vi "Flatten2DValues.vi"(9 "NumValues":u16[](array[numeric])=[1, 1, 1, 2, 4, 1], 10 "Values 2D":dbl[][](array[numeric])=[[1712710454.0, 9999.0], [0.0, 9999.0], [0.0, 9999.0], [1.0, 2.0], [9999.0, 9999.0], [9999.0, 9999.0]] format="%.2f", 11 "NumFrames":i32=6) -> (2 "Values 1D":dbl[](array[numeric]) format="%.2f")   [LabVIEW 2024]
panel:
  # "Takes a 2D array of values and flattens it to 1D.  Removes or adds extra\nelements based on NumValues.  The result is a 1D Values array of the\nexact size to hold all write and read data."
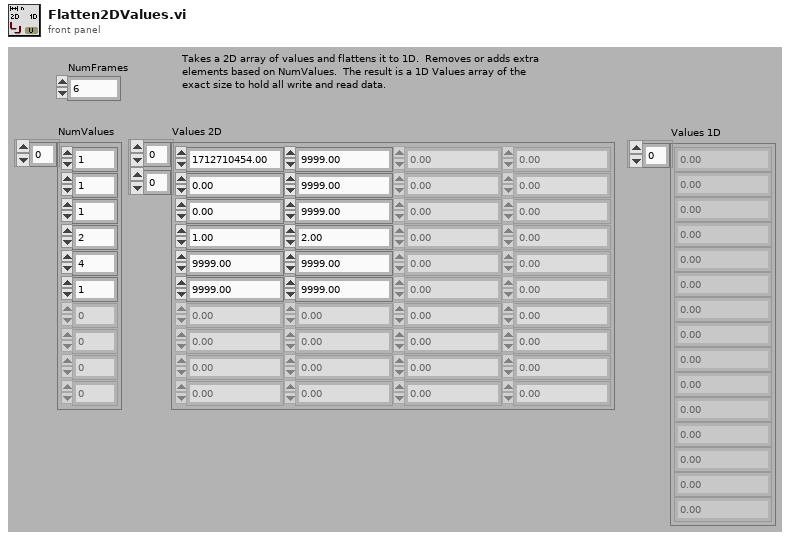
[diagram p1: front panel]
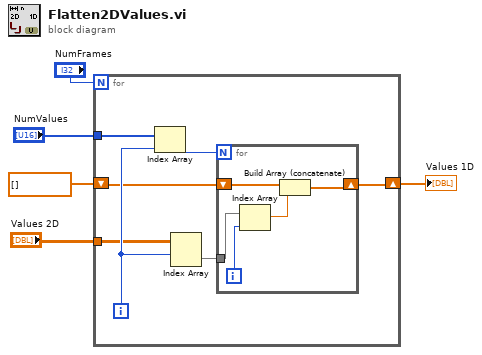
[diagram p0: block diagram]
diagram:
  n1 = for {
    N: "NumFrames" -> [_]
    shift-right: [w8] -> w3
    shift-left: dbl[] [] -> [w9]
    tunnel: "NumValues" -> [w7]
    tunnel: "Values 2D" -> [w6]
    i -> [w12]
    n2 = Index Array(array=w7, index=w12) -> (element=w10:u16)
    n3 = Index Array(array=w6, index (row)=w12) -> (element=w11:dbl[])  [unwired: 1 in]
    n4 = for {
      N: w10 -> [_]
      tunnel: w11 -> [w14]
      shift-right: [w17] -> w8
      shift-left: w9 -> [w16]
      i -> [w13]
      n5 = Index Array(array=w14, index=w13) -> (element=w15:dbl)
      n6 = Build Array (concatenate)(w16, w15) -> (w17:dbl[])
    }
  }
  "Values 1D" <- w3
